vi "Test_sqlite3ReadColumnWorks_ReturnsArray.vi"(8 "error in (no error)":errorcluster, 11 "TestCase in":refnum<class "Test sqlite3.lvclass">) -> (0 "error out":errorcluster, 3 "TestCase out":refnum<class "Test sqlite3.lvclass">)   [LabVIEW 2020, in "Test sqlite3.lvclass"]
uses:
  Test sqlite3.lvclass
  Test sqlite3.lvclass/Test sqlite3.ctl
  <vilib>/addons/_JKI Toolkits/VI Tester/TestCase.llb/TestCase.lvclass
  7035df59-fb91-4712-9474-277b58e51850.vi
  C:/Program Files/National Instruments/LabVIEW 2020/vi.lib/addons/_JKI Toolkits/VI Tester/TestCase.llb/TestCase.lvclass
  C:/Users/Fred.Guo/Desktop/Database-configuration/externals/database-interface/Test/Test sqlite3/Test sqlite3.lvclass
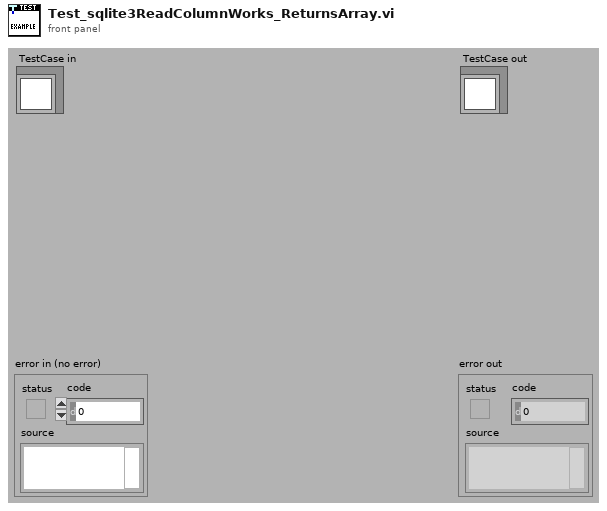
[diagram p1: front panel]
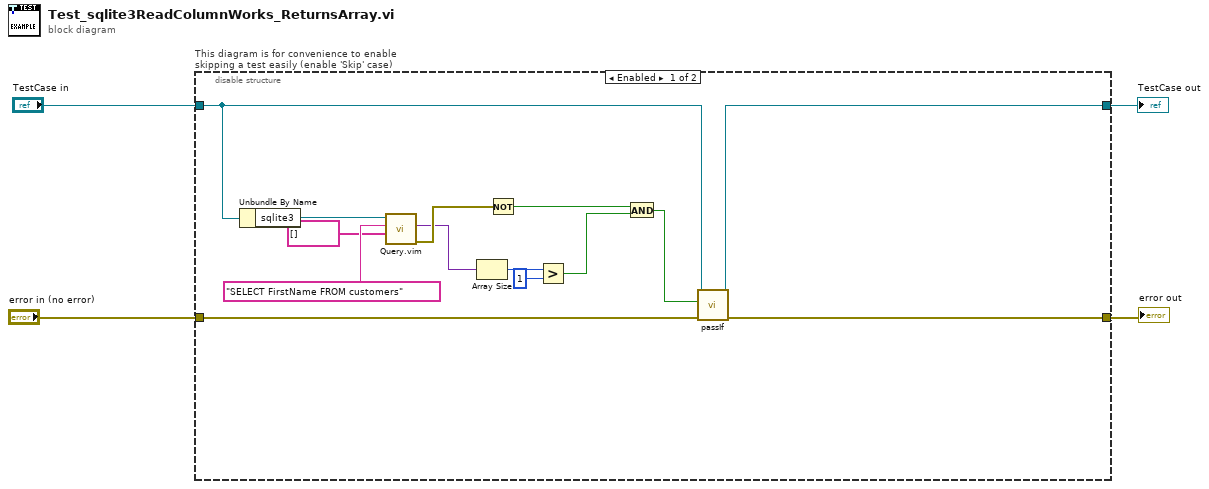
[diagram p0: block diagram]
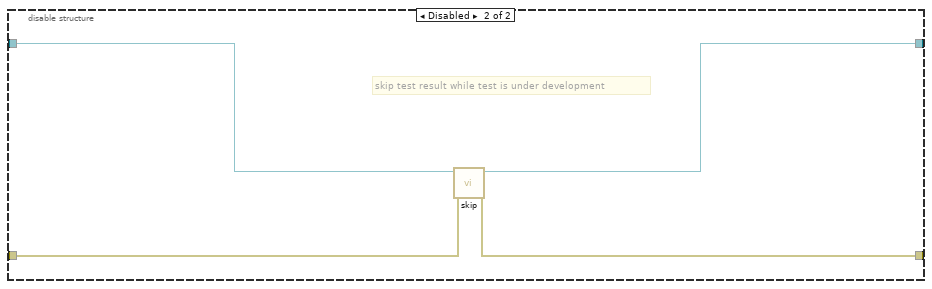
[diagram p2: hidden frame]
diagram:
  n1 = disable-structure "This diagram is for convenience to enable skipping a test easily (enable 'Skip' case)" shown="Enabled" {
    disable-tunnel: "TestCase in" -> [w16 w22]
    disable-tunnel: [w18 w20] -> w1
    disable-tunnel: [w17 w21] -> w3
    disable-tunnel: "error in (no error)" -> [w15 w19]
    frame Enabled {
      n2 = Unbundle By Name(w16) -> ("sqlite3"=w10:refnum<class "sqlite3.lvclass">)
      n3 = call "Query.vim"("Type and Default"=string[] [], "Query string"="SELECT FirstName FROM customers", "IDatabase in"=w10) -> ("error out"=w11:errorcluster, "Result"=w8:variant)  [unwired: 6 in, 1 out]
      n4 = Array Size(array=w8) -> (size(s)=w7:i32)
      n5 = Not(x=w11) -> (.not. x?=w14:bool)
      n6 = Greater?(x=w7, y=1) -> (0:w5:bool)
      n7 = And(x=w14, y=w5) -> (x .and. y?=w13:bool)
      n8 = call-dynamic "passIf.vi"("error in (no error)"=w15, "pass"=w13, "TestCase in"=w16) -> ("error out"=w17:errorcluster, "TestCase out"=w18:refnum<class "Test sqlite3.lvclass">)  [unwired: 7 in]
    }
    frame Disabled {
      # "skip test result while test is under development"
      n9 = call <vilib>:"skip.vi"("error in (no error)"=w19, "TestCase in"=w22) -> ("error out"=w21:errorcluster, "TestCase out"=w20:refnum<class "Test sqlite3.lvclass">)  [unwired: 8 in]
    }
  }
  "error out" <- w3
  "TestCase out" <- w1
